vi "To Integral Cycles.vi"(7 "reset? (F)":bool, 8 "error in (no error)":errorcluster, 10 "trigger information":T1={"trigger times [s]"=[], "triggers per cycle"=2}, 11 "data in":waveform(dbl)[](array[waveform])) -> (0 "error out":errorcluster, 3 "integral-cycle data":waveform(dbl)[](array[waveform]))   [LabVIEW 2016, in "NI_EP_Power Measurement.lvlib"]
doc: "Divides the voltage and current signals into integral-cycle data for power measurement, according to the trigger times that you specify."
uses:
  <vilib>/addons/Electrical Power/Power Measurement/NI_EP_Power Measurement.lvlib
  <vilib>/Waveform/WDTOps.llb/WDT Append Waveforms DBL.vi
  <vilib>/Waveform/WDTOps.llb/WDT Number of Waveform Samples DBL.vi
  <vilib>/Waveform/WDTOps.llb/WDT Get Waveform Subset DBL.vi
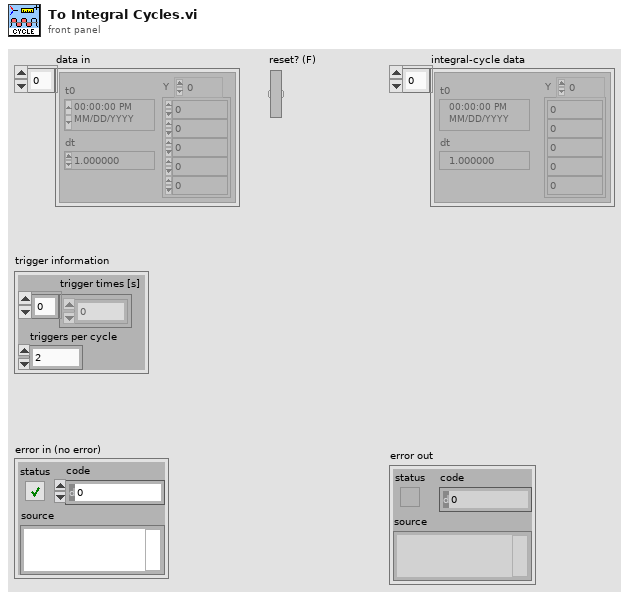
[diagram p1: front panel]
types:
  T1 = cluster{"trigger times [s]":dbl[], "triggers per cycle":u8}
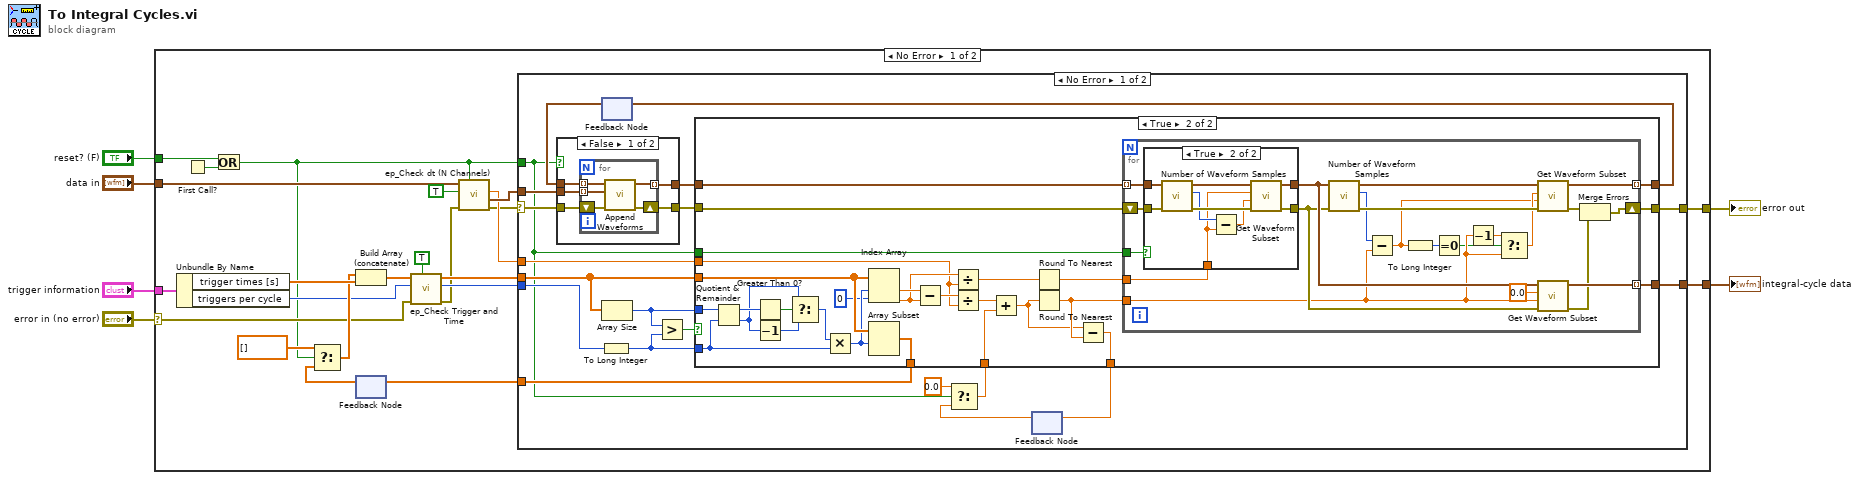
[diagram p0: block diagram]
diagram:
  n1 = case shown="No Error" "error in (no error)" {
    selector: "error in (no error)" -> [w9 w127]
    tunnel: "trigger information" -> [w27 _]
    tunnel: "data in" -> [w14 _]
    tunnel: "reset? (F)" -> [w28 _]
    tunnel: [w21 _] -> w5
    tunnel: [w15 w127] -> w4
    frame No Error {
      n2 = Unbundle By Name(w27) -> ("trigger times [s]"=w26:dbl[], "triggers per cycle"=w17:u8)
      n3 = First Call?() -> (First Call?: T/F=w29:bool)
      n4 = Or(x=w28, y=w29) -> (x .or. y?=w7:bool)
      n5 = feedback #1() -> (w22:dbl[])  [unwired: 1 in]
      n6 = Select(t=dbl[] [] ("trigger positions [s]"), s=w7, f=w22) -> (s? t:f=w24:dbl[])
      n7 = Build Array (concatenate)(w24, w26) -> (w20:dbl[])
      n8 = call <vilib>:"ep_Check Trigger and Time.vi"("trigger? (F)"=TRUE ("trigger? (T)"), "error in (no error)"=w9, "triggers per cycle"=w17, "trigger/positions [s]"=w20) -> ("error out"=w10:errorcluster, "dup triggers per cycle"=w18:u8, "dup trigger/positions [s]"=w19:dbl[])  [unwired: 5 in]
      n9 = call <vilib>:"ep_Check dt (N Channels).vi"("reset? (F)"=w7, "error in (no error)"=w10, "waveforms only? (F)"=TRUE, "waveforms"=w14) -> ("error out"=w11:errorcluster, "dup waveforms"=w13:waveform(dbl)[], "dt"=w12:dbl)  [unwired: 3 in, 2 out]
      n10 = case shown="No Error" w11 {
        selector: w11 -> [w40 w126]
        tunnel: [w49 _] -> w23
        tunnel: [w48 _] -> w21
        tunnel: w19 -> [w47 _]
        tunnel: w18 -> [w46 _]
        tunnel: w7 -> [w32 _]
        tunnel: w13 -> [w41 _]
        tunnel: [w36 w126] -> w15
        tunnel: w12 -> [w35 _]
        frame No Error {
          n11 = To Long Integer(number=w46) -> (32bit integer=w43:i32)
          n12 = feedback #2() -> (w37:waveform(dbl)[])  [unwired: 1 in]
          n13 = case shown="False" w32 {
            tunnel: w41 -> [w54 w60]
            tunnel: w40 -> [w53 w61]
            tunnel: [w52 w60] -> w39
            tunnel: [w51 w61] -> w38
            tunnel: w37 -> [w50 _]
            frame False {
              n14 = for {
                tunnel: w50 -> [w59] mode=indexing
                tunnel: w54 -> [w58] mode=indexing
                shift-right: [w56] -> w51
                shift-left: w53 -> [w57]
                tunnel: [w55] -> w52 mode=indexing
                n15 = call-poly <vilib>:"Append Waveforms.vi"("error in (no error)"=w57, "waveform B"=w58, "waveform A"=w59) -> ("error out"=w56:errorcluster, "waveform out"=w55:waveform(dbl))  [unwired: 7 in]
              }
            }
            frame True {
            }
          }
          n16 = Array Size(array=w47) -> (size(s)=w45:i32)
          n17 = Greater?(x=w45, y=w43) -> (0:w42:bool)
          n18 = feedback #3() -> (w33:dbl)  [unwired: 1 in]
          n19 = Select(t=0.0, s=w32, f=w33) -> (s? t:f=w30:dbl)
          n20 = case shown="True" w42 {
            tunnel: w47 -> [w65 w92]
            tunnel: w43 -> [_ w89]
            tunnel: w45 -> [_ w93]
            tunnel: [w65 w91] -> w49
            tunnel: [w64 w78] -> w44
            tunnel: [_ w79] -> w48
            tunnel: w32 -> [_ w81]
            tunnel: w39 -> [w64 w73]
            tunnel: w38 -> [w63 w80]
            tunnel: [w63 w77] -> w36
            tunnel: w35 -> [_ w71]
            tunnel: [w62 w70] -> w34
            tunnel: w30 -> [w62 w69]
            frame False {
            }
            frame True {
              n21 = Quotient & Remainder(x=w93, y=w89) -> (x-y*floor(x/y)=w90:i32, floor(x/y)=w86:i32)
              n22 = Greater Than 0?(x=w90) -> (x > 0?=w88:bool)
              n23 = Decrement(x=w86) -> (x-1=w82:i32)
              n24 = Select(t=w86, s=w88, f=w82) -> (s? t:f=w87:i32)
              n25 = Multiply(x=w87, y=w89) -> (x*y=w85:i32)
              n26 = Index Array(array=w92, index #1=w85, index #2=0 ("index")) -> (element #1=w84:dbl, element #2=w74:dbl)
              n27 = Array Subset(array=w92, index=w85) -> (w91:dbl[])  [unwired: 1 in]
              n28 = Subtract(x=w84, y=w74) -> (x-y=w76:dbl)
              n29 = Divide(x=w74, y=w71) -> (x/y=w75:dbl)
              n30 = Divide(x=w76, y=w71) -> (x/y=w67:dbl)
              n31 = Add(x=w67, y=w69) -> (x+y=w66:dbl)
              n32 = Round To Nearest(number=w75) -> (nearest integer value=w72:dbl)
              n33 = Round To Nearest(number=w66) -> (nearest integer value=w68:dbl)
              n34 = Subtract(x=w66, y=w68) -> (x-y=w70:dbl)
              n35 = for {
                tunnel: w73 -> [w114] mode=indexing
                tunnel: w81 -> [w113]
                shift-right: [w103] -> w77
                shift-left: w80 -> [w112]
                tunnel: [w111] -> w79 mode=indexing
                tunnel: [w104] -> w78 mode=indexing
                tunnel: w72 -> [w101]
                tunnel: w68 -> [w97]
                n36 = case shown="True" w113 {
                  tunnel: w114 -> [w116 w125]
                  tunnel: w112 -> [w115 w123]
                  tunnel: [w116 w121] -> w107
                  tunnel: [w115 w120] -> w105
                  tunnel: w101 -> [_ w118]
                  frame False {
                  }
                  frame True {
                    n37 = call-poly <vilib>:"Number of Waveform Samples.vi"("error in (no error)"=w123, "waveform in"=w125) -> ("error out"=w122:errorcluster, "number of samples"=w119:i32, "waveform out"=w124:waveform(dbl))  [unwired: 7 in]
                    n38 = Subtract(x=w119, y=w118) -> (x-y=w117:dbl)
                    n39 = call-poly <vilib>:"Get Waveform Subset.vi"("error in (no error)"=w122, "duration"=w117, "start samples/time"=w118, "waveform in"=w124) -> ("error out"=w120:errorcluster, "waveform out"=w121:waveform(dbl))  [unwired: 2 in, 2 out]
                  }
                }
                n40 = call-poly <vilib>:"Number of Waveform Samples.vi"("error in (no error)"=w105, "waveform in"=w107) -> ("error out"=w108:errorcluster, "number of samples"=w100:i32, "waveform out"=w109:waveform(dbl))  [unwired: 7 in]
                n41 = Subtract(x=w100, y=w97) -> (x-y=w96:dbl)
                n42 = To Long Integer(number=w96) -> (32bit integer=w94:i32)
                n43 = Equal To 0?(x=w94) -> (x = 0?=w95:bool)
                n44 = Decrement(x=w97) -> (x-1=w98:dbl)
                n45 = Select(t=w98, s=w95, f=w97) -> (s? t:f=w99:dbl)
                n46 = call-poly <vilib>:"Get Waveform Subset.vi"("error in (no error)"=w108, "duration"=w96, "start samples/time"=w99, "waveform in"=w109) -> ("error out"=w110:errorcluster, "waveform out"=w104:waveform(dbl))  [unwired: 2 in, 2 out]
                n47 = call-poly <vilib>:"Get Waveform Subset.vi"("error in (no error)"=w105, "duration"=w97, "start samples/time"=0.0, "waveform in"=w107) -> ("error out"=w102:errorcluster, "waveform out"=w111:waveform(dbl))  [unwired: 2 in, 2 out]
                n48 = Merge Errors(w110, w102) -> (w103:errorcluster)
              }
            }
          }
          n49 = feedback-in #2(w44) -> ()
          n50 = feedback-in #3(w34) -> ()
        }
        frame Error {
        }
      }
      n51 = feedback-in #1(w23) -> ()
    }
    frame Error {
    }
  }
  "error out" <- w4
  "integral-cycle data" <- w5
